vi "Average PSD.vi"() -> ()   [LabVIEW 2023]
doc: "This example shows how to continuously average the estimated power spectral density (PSD) of a univariate time series with the TSA Average PSD VI.\n\n<b>Instructions:</b>\n1) Run this VI.\n2) Try different averaging parameters.\n3) Observe the power spectral density of the signal."
uses:
  <vilib>/addons/Time Series Analysis/Utilities.llb/TSA Scale to EU (Single-Channel).vi
  <vilib>/addons/Time Series Analysis/Correlation and Spectral Analysis.llb/TSA Periodogram (Waveform).vi
  <vilib>/addons/_Advanced Signal Processing/NI_AdvSigProcTSA.lvlib
  <vilib>/measure/NI_MABase.lvlib
panel:
  in  "Averaging Parameters":T1={"Averaging Mode"=0, "Weighting Mode"=0, "Number of Averages"=10} {"Number of Averages" min=1; "Weighting Mode" items=["Linear", "Exponential"]; "Averaging Mode" items=["No averaging", "RMS averaging", "Peak hold"]}
  in  "stop":bool
  in  "dB on? (T)":bool=TRUE
  in  "Amplitude":dbl=1.0 format="%.2p"
  in  "Frequency":dbl=100.0 format="%.2p"
  in  "Sampling info":cluster{"Fs":dbl, "#s":dbl}={"Fs"=1000.0, "#s"=2000.0}
  in  "Channel info":T2={"Sensor Sensitivity (mV/EU)"=1000.0, "Engineering Units"=0, "Custom Label"="EU"} {"Engineering Units" items=["custom..."=0, "V"=1, "N"=20, "Pa"=2, "m/s^2"=4, "m/s"=5, "m"=6, "rad/s^2"=16, "rad/s"=17, "rad"=18]; "Sensor Sensitivity (mV/EU)" format="%.2f"}
  out "Completed averages":u32=980
  out "Averaging Done?":bool=TRUE
  in  "Window":u16(ring) items=["None ", "Hanning", "Hamming", "Blackman-Harris", "Exact Blackman", "Blackman", "Flat Top", "4 Term B-Harris ", "7 Term B-Harris", "Low Sidelobe"]
  in  "Frequency bins":i32=1024
  in  "reset":bool
  out "Power Spectral Density":cluster{"f0":dbl, "df":dbl, "S(f)":dbl[]}(graph)
  # "Overview: Shows how to continuously average the estimated power spectral density (PSD) of a univariate time series with the TSA Average PSD VI.\nRequirements: LabVIEW Full Development System, Advanced Signal Processing Toolkit\nInstructions: \n1. Run this VI.\n2. Try different averaging parameters.\n3. Observe the power spectral density of the signal. \n4. Click Stop to stop the VI."
  # "Simulated Signal"
  # "Periodogram Settings"
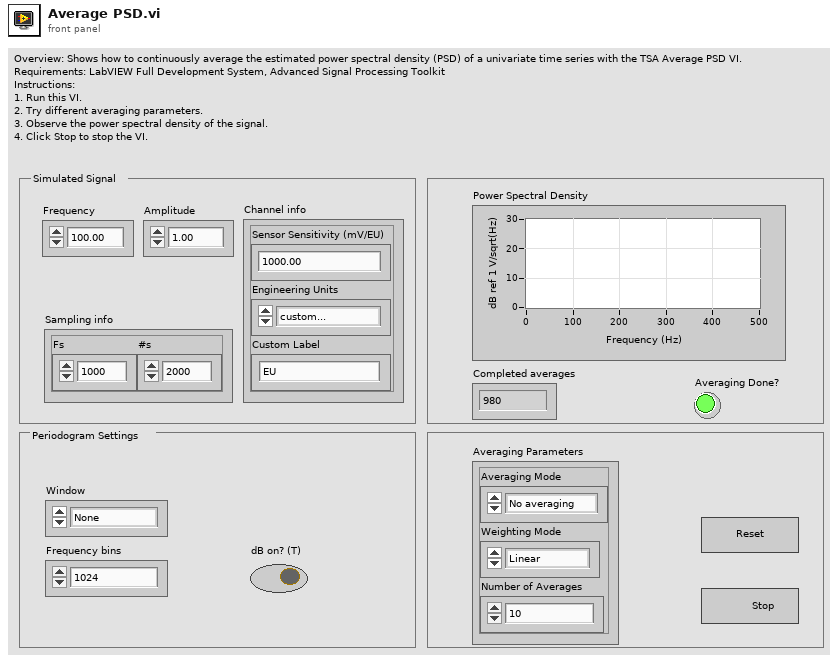
[diagram p1: front panel]
types:
  T1 = cluster{"Averaging Mode":u16, "Weighting Mode":u16, "Number of Averages":u32}
  T2 = cluster{"Sensor Sensitivity (mV/EU)":dbl, "Engineering Units":u16, "Custom Label":string}
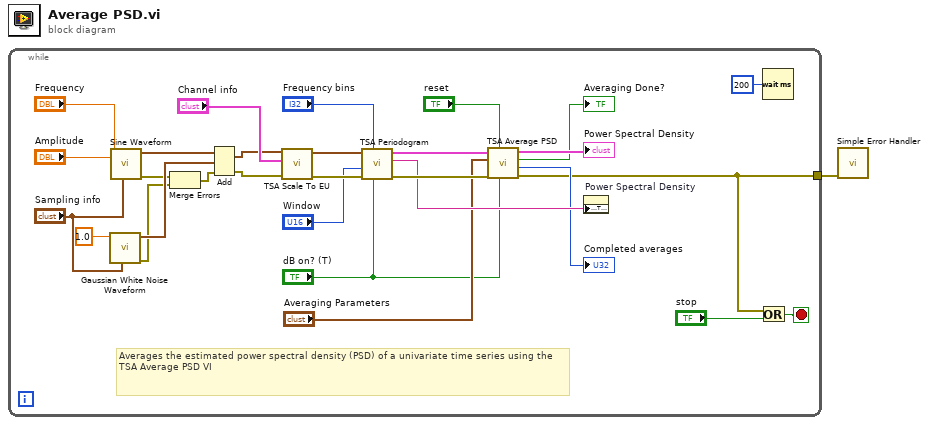
[diagram p0: block diagram]
diagram:
  n1 = while {
    tunnel: [w3] -> w1
    stop <- w2 stop-if-true
    # "Averages the estimated power spectral density (PSD) of a univariate time series using the TSA Average PSD VI"
    n2 = call <vilib>:"Gaussian White Noise Waveform.vi"("sampling info"="Sampling info", "standard deviation"=1.0) -> ("error out"=w7:errorcluster, "signal out"=w17:waveform(dbl))  [unwired: 3 in, 5 out]
    n3 = call <vilib>:"Sine Waveform.vi"("sampling info"="Sampling info", "amplitude"="Amplitude", "frequency"="Frequency") -> ("error out"=w8:errorcluster, "signal out"=w18:waveform(dbl))  [unwired: 4 in, 3 out]
    n4 = Merge Errors(w8, w7) -> (w6:errorcluster)
    n5 = Add(1:w17, 2:w18, 4:w6) -> (0:w19:waveform(dbl), 3:w5:errorcluster)
    n6 = call-poly <vilib>:"TSA Scale To EU.vi"("error in (no error)"=w5, "scale info"="Channel info", "Xt"=w19) -> ("error out"=w26:errorcluster, "Xt out"=w27:waveform(dbl))  [unwired: 7 out]
    n7 = call-poly <vilib>:"TSA Periodogram.vi"("dB on? (T)"="dB on? (T)", "frequency bins"="Frequency bins", "error in (no error)"=w26, "window"="Window", "Xt"=w27) -> ("error out"=w29:errorcluster, "unit"=w24:string, "PSD"=w30:cluster{"f0":dbl, "df":dbl, "S(f)":dbl[]})  [unwired: 4 out]
    n8 = call <vilib>:"TSA Average PSD.vi"("dB on? (T)"="dB on? (T)", "reset? (F)"="reset", "error in (no error)"=w29, "averaging parameters"="Averaging Parameters", "PSD"=w30) -> ("error out"=w3:errorcluster, "completed averages"=→"Completed averages":u32, "averaging done"=→"Averaging Done?":bool, "PSD averaged"=→"Power Spectral Density":cluster{"f0":dbl, "df":dbl, "S(f)":dbl[]})  [unwired: 3 out]
    n9 = property on="Power Spectral Density" class="WFGraph (strict)"("Y Scale.Name Label.Text"=w24) -> ()  [unwired: 2 in, 2 out]
    n10 = Or(x=w3, y="stop") -> (x .or. y?=w2:bool)
    n11 = Wait (ms)(milliseconds to wait=u32 200 ("millisecond multiple")) -> ()  [unwired: 1 out]
  }
  n12 = call <vilib>:"Simple Error Handler.vi"("error in (no error)"=w1) -> ()  [unwired: 4 in, 5 out]
